vi "lsl get version.vi"(8 "error in":errorcluster, 11 "streaminfo":T1) -> (0 "error out":errorcluster, 3 "version":i32)   [LabVIEW 2016, in "Lab Streaming Layer.lvlib"]
doc: "extern LIBLSL_C_API int32_t lsl_get_version(lsl_streaminfo info);"
uses:
  Lab Streaming Layer.lvlib
  Custom Controls/lsl_streaminfo.ctl
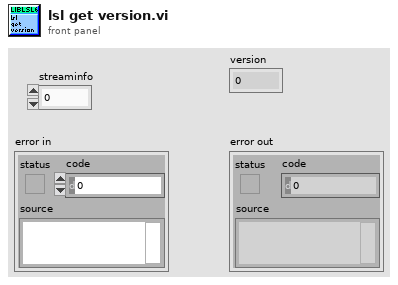
[diagram p1: front panel]
types:
  T1 = typedef "Lab Streaming Layer.lvlib/lsl_streaminfo.ctl" = u64
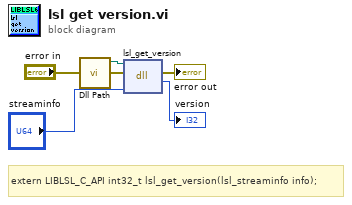
[diagram p0: block diagram]
diagram:
  # "extern LIBLSL_C_API int32_t lsl_get_version(lsl_streaminfo info);"
  n1 = call "Dll Path.vi"() -> ("Dll path"=w1:path)  [unwired: 11 in]
  n2 = dll-call lib="E:/LabStreamingLayer/liblsl-LabVIEW-master/liblsl-LabVIEW-master/lsl.dll" fn="lsl_get_version"(path in=w1, error in="error in", "info"="streaminfo") -> (error out=→"error out":errorcluster, "return type"=→"version":i32)  [unwired: 2 in, 1 out]
